vi "MoveFileToProcessedFolder.vi"(8 "error in (no error)":errorcluster, 11 "source file":path) -> (0 "error out":errorcluster, 3 "new path":path)   [LabVIEW 2016, in "VCL_2_DSC.lvclass"]
uses:
  VCL_2_DSC.lvclass
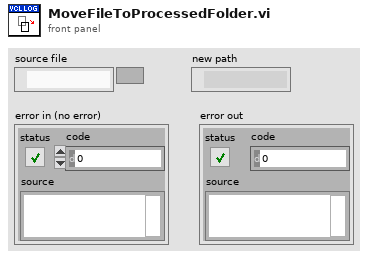
[diagram p1: front panel]
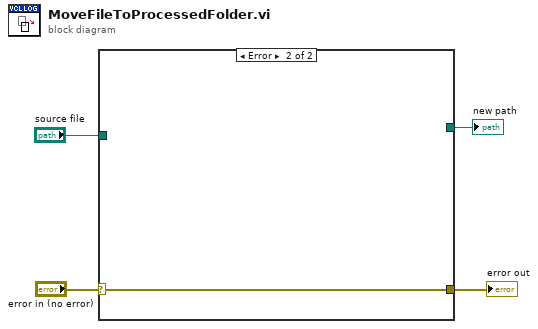
[diagram p0: block diagram]
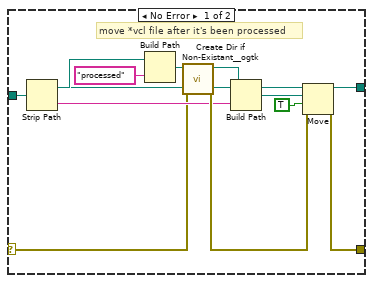
[diagram p2: hidden frame]
diagram:
  n1 = case shown="Error" "error in (no error)" {
    selector: "error in (no error)" -> [w5 w17]
    tunnel: [w8 _] -> w4
    tunnel: "source file" -> [w7 _]
    tunnel: [w16 w17] -> w1
    frame No Error {
      # "move *vcl file after it's been processed"
      n2 = Strip Path(path=w7) -> (stripped path=w12:path, name=w11:string)
      n3 = Build Path(base path=w12, name or relative path="processed") -> (appended path=w10:path)
      n4 = call <userlib>:"Create Dir if Non-Existant__ogtk.vi"("error in (no error)"=w5, "Directory Path"=w10) -> ("error out"=w15:errorcluster, "dup Directory Path"=w6:path)  [unwired: 7 in, 1 out]
      n5 = Build Path(base path=w6, name or relative path=w11) -> (appended path=w14:path)
      n6 = Move(source path=w7, error in=w15, 9:TRUE ("overwrite (F)"), 10:w14) -> (error out=w16:errorcluster, 3:w8:path)  [unwired: 1 in, 1 out]
    }
    frame Error {
    }
  }
  "error out" <- w1
  "new path" <- w4
